vi "Get Settings.vi"(8 "error in (no error)":errorcluster, 11 "LogEngine":refnum<class "LogEngine.lvclass">) -> (0 "error out":errorcluster, 2 "LogEngine Settings":T1, 3 "LogEngine out":refnum<class "LogEngine.lvclass">)   [LabVIEW 2017, in "LogEngine.lvclass"]
doc: "Developed by Kevin Thompson\nkevin@thompsonengineering.net\n\nCopyright 2018-2020\nThompson Engineering, LLC"
uses:
  LogEngine.lvclass
  Data Types/TD LogEngine Settings--cluster.ctl
  LogEngine.lvclass/LogEngine.ctl
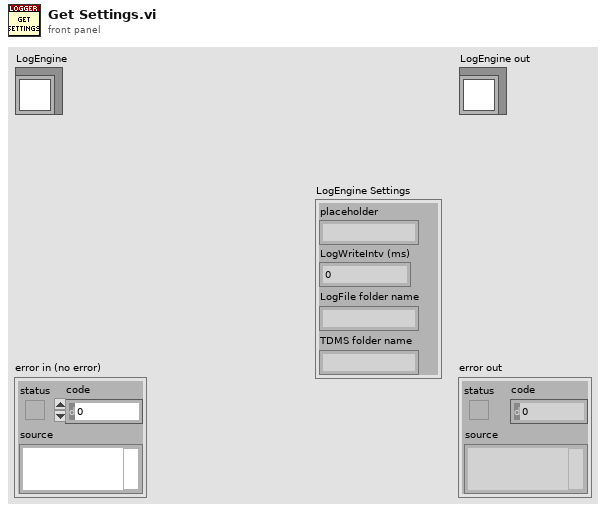
[diagram p1: front panel]
types:
  T1 = typedef "LogEngine.lvclass/TD LogEngine Settings--cluster.ctl" = cluster{"placeholder":string, "LogWriteIntv (ms)":u32, "LogFile folder name":string, "TDMS folder name":string}
  T2 = typedef "LogEngine.lvclass/TD Obj Data_LogEngine.ctl" = cluster{"LogEngine Settings":T1, "Logger State Data":T3, "tdms fileref":refnum<k34>, "LogHeaderData":T5, "LogHeaderString":string}
  T3 = typedef "LogEngine.lvclass/TD Logger State Data--cluster.ctl" = cluster{"Logger State":T4, "TDMS Logging State":T4, "LogFile path":path, "TDMS File path":path, "vData":variant}
  T4 = typedef "LogEngine.lvclass/TD Logger State--enum.ctl" = enum16{"Unknown", "Logging", "NotLogging", "Error"}
  T5 = typedef "LogEngine.lvclass/LogHeaderData--cluster.ctl" = cluster{"SessionSettings":T6, "SequenceFile":string, "SeqFileParams":T7, "AI TaskName":string, "SamplingRate":dbl, "SamplesPerAcq":i32}
  T6 = typedef "SessionSettings--cluster.ctl" = cluster{"Job_ID":string, "Operator_ID":string, "Station_ID":string, "Job_Description":string}
  T7 = typedef "Sequencer.lvclass/SeqFileParameters--cluster.ctl" = cluster{"MotorVel":dbl, "VoltageSP":dbl, "MoveSF":dbl, "IntegTime":dbl, "Pgain":dbl, "Igain":dbl, "Dgain":dbl, "PosMode":T8, "OscMode":T9, "WeldCurSF":dbl}
  T8 = typedef "Sequencer.lvclass/SeqFileParam_PosMode--enum.ctl" = enum16{"NORM", "ABS", "HYBRID"}
  T9 = typedef "Sequencer.lvclass/SeqFileParam_OscMode--enum.ctl" = enum16{"OFF", "ON"}
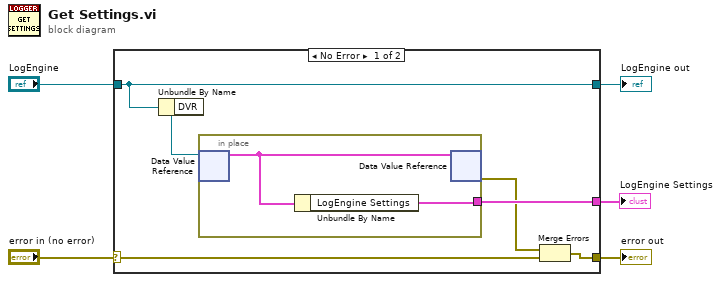
[diagram p0: block diagram]
diagram:
  n1 = case shown="No Error" "error in (no error)" {
    selector: "error in (no error)" -> [w11 w14]
    tunnel: [w7 w14] -> w4
    tunnel: [w10 w15] -> w2
    tunnel: "LogEngine" -> [w10 w15]
    tunnel: [w8 _] -> w1
    frame No Error {
      n2 = Unbundle By Name(w10) -> ("DVR"=w9:refnum<data-value>)
      n3 = in-place {
        in-place-border: [w12] -> w8
        n4 = in-place-dvr #1(w9) -> (w13:T2)  [unwired: 1 out]
        n5 = Unbundle By Name(w13) -> ("LogEngine Settings"=w12:T1)
        n6 = in-place-dvr #1(w13) -> (w6:errorcluster)  [unwired: 1 out]
      }
      n7 = Merge Errors(w6, w11) -> (w7:errorcluster)
    }
    frame Error {
    }
  }
  "error out" <- w4
  "LogEngine out" <- w2
  "LogEngine Settings" <- w1
